vi "Speed conversion.vi"(11 "Filtered data":i32) -> (3 "Numeric":sgl)   [LabVIEW 2016]
uses:
  <vilib>/rvi/FXPMathLib/FxpDiv/subVIs/nifxpmath_Div_SimConfig.ctl
  <vilib>/rvi/FXPMathLib/FxpDiv/simVIs/DllFxpDivTemp_sub.vi
  <vilib>/rvi/FXPMathLib/FxpDiv/XNode/nifxpmath_Div.xnode
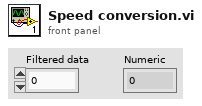
[diagram p1: front panel]
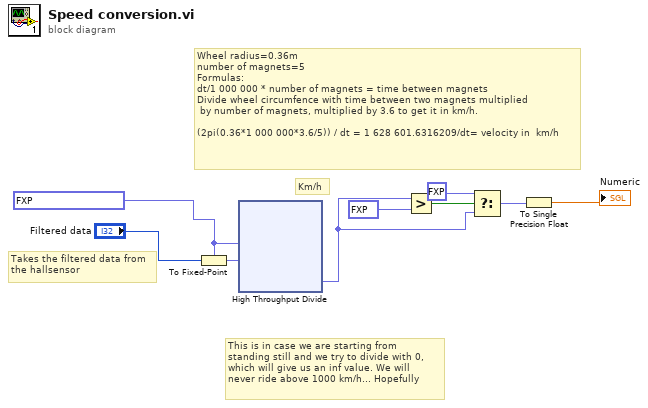
[diagram p0: block diagram]
diagram:
  w1 = fxp<+,32,21> 1628601.6318359375 ("x")
  # "Takes the filtered data from\nthe hallsensor"
  # "Wheel radius=0.36m\nnumber of magnets=5\nFormulas:\ndt/1 000 000 * number of magnets = time between magnets\nDivide wheel circumfence with time between two magnets multiplied\n by number of magnets, multiplied by 3.6 to get it in km/h.\n\n(2pi(0.36*1 000 000*3.6/5)) / dt = 1 628 601.6316209/dt= velocity in  km/h"
  # "This is in case we are starting from\nstanding still and we try to divide with 0, \nwhich will give us an inf value. We will \nnever ride above 1000 km/h... Hopefully"
  # "Km/h"
  n1 = To Fixed-Point(fixed-point type=w1, number="Filtered data") -> (fixed-point=w2:fxp<+,32,21>)
  n2 = xnode "High Throughput Divide"("x"=w1, "y"=w2) -> ("x/y"=w3:fxp<+,32,32>)
  n3 = Greater?(x=w3, y=fxp<+,7,10> 1000.0) -> (0:w5:bool)
  n4 = Select(t=fxp<+,1,1> 0.0, s=w5, f=w3) -> (s? t:f=w7:fxp<+,32,32>)
  n5 = To Single Precision Float(number=w7) -> (single precision float=→"Numeric":sgl)
